vi "Assignment6.vi"() -> ()   [LabVIEW 2021]
panel:
  out "amber":bool
  out "green":bool
  out "red":bool
  in  "Stop":bool
  out "Counter":dbl
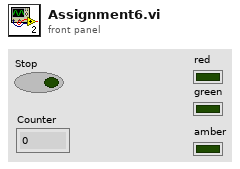
[diagram p1: front panel]
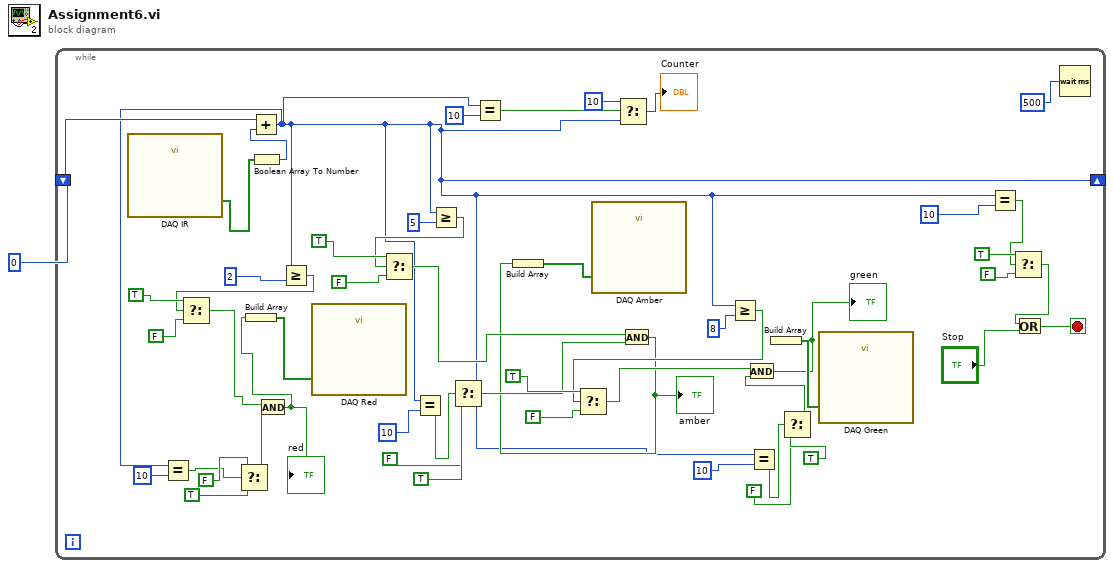
[diagram p0: block diagram]
diagram:
  n1 = while {
    shift-right: [w6] -> _
    shift-left: 0 -> [w53]
    stop <- w33 stop-if-true
    n2 = call "DAQ IR"() -> ("data"=w52:bool[])  [unwired: 17 in, 2 out]
    n3 = Boolean Array To Number(Boolean array=w52) -> (number=w48:u32)
    n4 = Add(x=w53, y=w48) -> (x+y=w6:u32)
    n5 = Equal?(x=w6, y=10) -> (x = y?=w4:bool)
    n6 = Select(t=FALSE, s=w4, f=TRUE) -> (s? t:f=w27:bool)
    n7 = Greater Or Equal?(x=w6, y=u32 2) -> (x >= y?=w30:bool)
    n8 = Select(t=TRUE, s=w30, f=FALSE) -> (s? t:f=w26:bool)
    n9 = And(x=w26, y=w27) -> (x .and. y?=w8:bool)
    "red" <- w8
    n10 = Build Array(w8) -> (w46:bool[])
    n11 = call "DAQ Red"("data"=w46) -> ()  [unwired: 17 in, 2 out]
    n12 = Equal?(x=w6, y=10) -> (x = y?=w25:bool)
    n13 = Greater Or Equal?(x=w6, y=u32 5) -> (x >= y?=w42:bool)
    n14 = Select(t=TRUE, s=w42, f=FALSE) -> (s? t:f=w22:bool)
    n15 = Select(t=FALSE, s=w25, f=TRUE) -> (s? t:f=w21:bool)
    n16 = Equal?(x=w6, y=u32 10) -> (x = y?=w12:bool)
    n17 = Select(t=u32 10, s=w12, f=w6) -> (s? t:f=→"Counter":u32)
    n18 = And(x=w22, y=w21) -> (x .and. y?=w10:bool)
    "amber" <- w10
    n19 = Build Array(w10) -> (w20:bool[])
    n20 = call "DAQ Amber"("data"=w20) -> ()  [unwired: 17 in, 2 out]
    n21 = Greater Or Equal?(x=w6, y=u32 8) -> (x >= y?=w38:bool)
    n22 = Select(t=TRUE, s=w38, f=FALSE) -> (s? t:f=w16:bool)
    n23 = Equal?(x=w6, y=10) -> (x = y?=w19:bool)
    n24 = Select(t=FALSE, s=w19, f=TRUE) -> (s? t:f=w15:bool)
    n25 = And(x=w16, y=w15) -> (x .and. y?=w9:bool)
    "green" <- w9
    n26 = Build Array(w9) -> (w14:bool[])
    n27 = call "DAQ Green"("data"=w14) -> ()  [unwired: 17 in, 2 out]
    n28 = Equal?(x=w6, y=u32 10) -> (x = y?=w31:bool)
    n29 = Select(t=TRUE, s=w31, f=FALSE) -> (s? t:f=w32:bool)
    n30 = Or(x=w32, y="Stop") -> (x .or. y?=w33:bool)
    n31 = Wait (ms)(milliseconds to wait=u32 500) -> ()  [unwired: 1 out]
  }
